vi "Tosca-Visual Display TCP Server.vi"(0 "Address":string, 7 "Port":i32, 11 "Queue":refnum<queue>) -> (15 "No Error":errorcluster)   [LabVIEW 2020]
uses:
  Tosca-Visual Display Queue Data.ctl
  Tosca-Visual Display Action.ctl
  Tosca-Grating.ctl
  Tosca-Grating Type.ctl
panel:
  out "date/time string":string
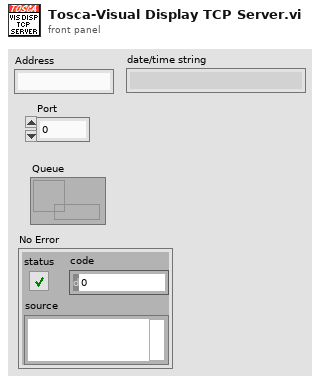
[diagram p1: front panel]
types:
  T1 = typedef "Tosca-Visual Display Queue Data.ctl" = cluster{"Action":T2, "Grating":T3}
  T2 = typedef "Tosca-Visual Display Action.ctl" = enum16{"NOOP", "Quit", "Buffer", "Draw", "Clear"}
  T3 = typedef "Tosca-Grating.ctl" = cluster{"Type":T4, "Orientation (deg)":dbl, "Spatial frequency (cpd)":dbl, "Velocity (Hz)":dbl, "Contrast":dbl, "Background intensity":dbl, "Duration (ms)":dbl, "Phase (cycles)":dbl}
  T4 = typedef "Tosca-Grating Type.ctl" = enum16{"OFF", "Square", "Sine"}
  T5 = cluster{"Grating type":T4, dbl, dbl, dbl, dbl, dbl, dbl, dbl}
  T6 = cluster{"Action":T2, cluster{"Grating type":T4, dbl, dbl, dbl, dbl, dbl, dbl, dbl}}
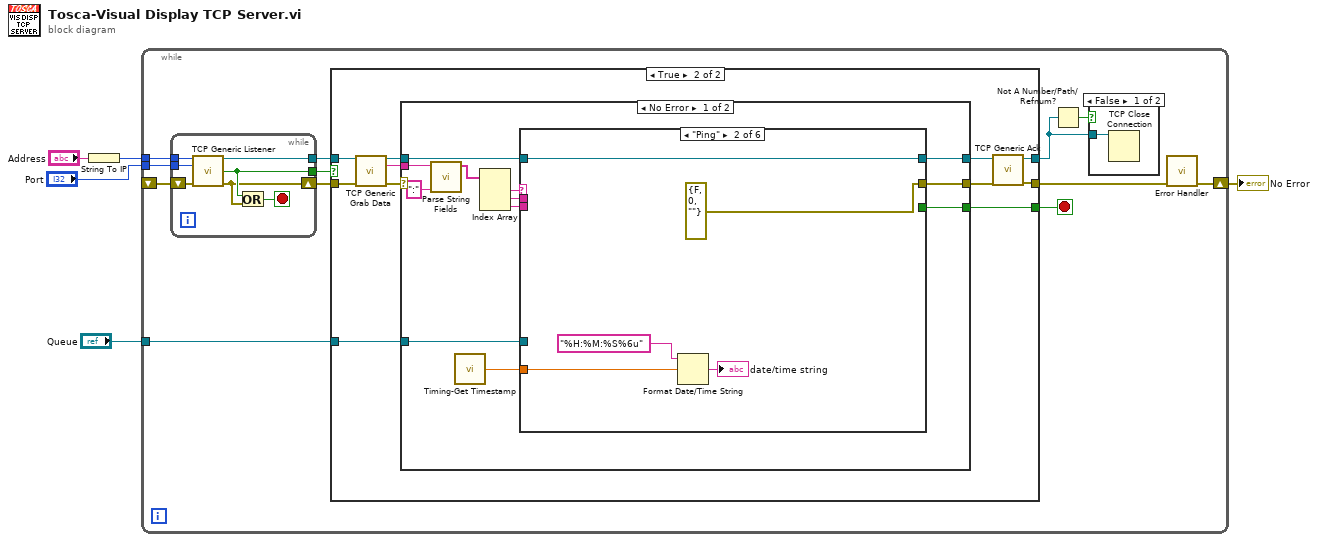
[diagram p0: block diagram]
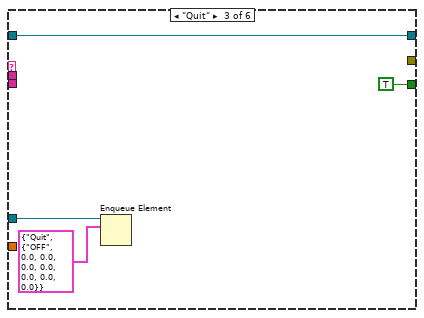
[diagram p5: hidden frame]
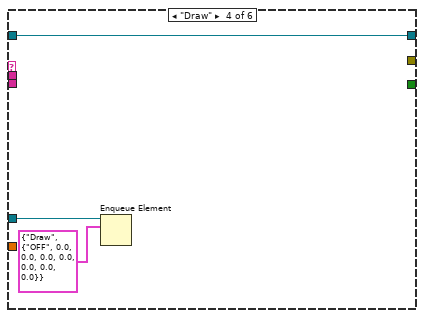
[diagram p6: hidden frame]
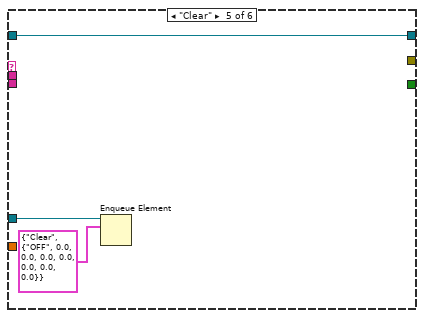
[diagram p7: hidden frame]
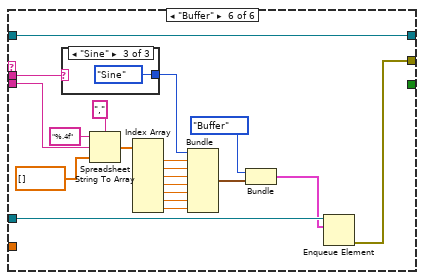
[diagram p8: hidden frame]
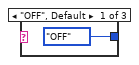
[diagram p9: hidden frame]
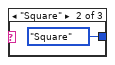
[diagram p10: hidden frame]
diagram:
  n1 = String To IP(1:"Address") -> (0:w4:u32)
  n2 = while {
    tunnel: w4 -> [w17]
    tunnel: "Port" -> [w16]
    shift-right: [w8] -> w2
    shift-left: _ -> [w15]
    tunnel: "Queue" -> [w6]
    stop <- w7 stop-if-true
    n3 = while {
      tunnel: w17 -> [w91]
      tunnel: w16 -> [w90]
      shift-right: [w86] -> w14
      shift-left: w15 -> [w89]
      tunnel: [w87] -> w13
      tunnel: [w88] -> w12
      stop <- w85 stop-if-true
      n4 = call "TCP Generic Listener.vi"("net address"=w91, "port"=w90, "error in (no error)"=w89) -> ("connection ID"=w88:refnum<k5>, "Connected?"=w87:bool, "error out"=w86:errorcluster)  [unwired: 10 in]
      n5 = Or(x=w87, y=w86) -> (x .or. y?=w85:bool)
    }
    n6 = case shown="True" w13 {
      tunnel: w14 -> [w19 w21]
      tunnel: w12 -> [w20 w31]
      tunnel: [w20 w25] -> w10
      tunnel: [w19 w24] -> w9
      tunnel: [_ w23] -> w7
      tunnel: w6 -> [_ w22]
      frame False {
      }
      frame True {
        n7 = call "TCP Generic Grab Data.vi"("connection ID"=w31, "error in (no error)"=w21) -> ("connection ID out"=w28:refnum<k5>, "data out"=w30:string, "error out"=w29:errorcluster)  [unwired: 11 in]
        n8 = case shown="No Error" w29 {
          selector: w29 -> [_ w83]
          tunnel: w30 -> [w43 _]
          tunnel: w28 -> [w42 w84]
          tunnel: [w39 w84] -> w27
          tunnel: [w38 w83] -> w26
          tunnel: [w37 _] -> w23
          tunnel: w22 -> [w33 _]
          frame No Error {
            n9 = call "Parse String Fields.vi"("Separator"=":", "String"=w43) -> ("Fields"=w41:string[])  [unwired: 8 in, 1 out]
            n10 = call "Timing-Get Timestamp.vi"() -> ("double precision float"=w32:dbl)  [unwired: 14 in, 1 out]
            n11 = Index Array(array=w41) -> (element #1=w40:string, element #2=w36:string, element #3=w35:string)  [unwired: 3 in]
            n12 = case shown="\"Ping\"" w40 {
              tunnel: w42 -> [w44 w49 w53 w56 w59 w79]
              tunnel: [w44 w49 w53 w56 w59 w79] -> w39
              tunnel: [_ errorcluster {"status"=FALSE, "code"=0, "source"=""} ("error constant") _ _ _ w77] -> w38
              tunnel: [_ _ TRUE _ _ _] -> w37
              tunnel: w36 -> [_ _ _ _ _ w73]
              tunnel: w35 -> [_ _ _ _ _ w76]
              tunnel: w33 -> [_ _ w51 w55 w58 w78]
              tunnel: w32 -> [_ w45 _ _ _ _]
              frame "", Default {
              }
              frame "Ping" {
                n13 = Format Date/Time String(time format string (%c)="%H:%M:%S%6u", seconds (now)=w45) -> (date/time string=→"date/time string":string)  [unwired: 1 in]
              }
              frame "Quit" {
                n14 = Enqueue Element(queue=w51, element=T1 {"Action"=enum."Quit", "Grating"={"Type"=enum."OFF", "Orientation (deg)"=0.0, "Spatial frequency (cpd)"=0.0, "Velocity (Hz)"=0.0, "Contrast"=0.0, "Background intensity"=0.0, "Duration (ms)"=0.0, "Phase (cycles)"=0.0}} ("Queue Data")) -> ()  [unwired: 2 in, 3 out]
              }
              frame "Draw" {
                n15 = Enqueue Element(queue=w55, element=T1 {"Action"=enum."Draw", "Grating"={"Type"=enum."OFF", "Orientation (deg)"=0.0, "Spatial frequency (cpd)"=0.0, "Velocity (Hz)"=0.0, "Contrast"=0.0, "Background intensity"=0.0, "Duration (ms)"=0.0, "Phase (cycles)"=0.0}} ("Queue Data")) -> ()  [unwired: 2 in, 3 out]
              }
              frame "Clear" {
                n16 = Enqueue Element(queue=w58, element=T1 {"Action"=enum."Clear", "Grating"={"Type"=enum."OFF", "Orientation (deg)"=0.0, "Spatial frequency (cpd)"=0.0, "Velocity (Hz)"=0.0, "Contrast"=0.0, "Background intensity"=0.0, "Duration (ms)"=0.0, "Phase (cycles)"=0.0}} ("Queue Data")) -> ()  [unwired: 2 in, 3 out]
              }
              frame "Buffer" {
                n17 = case shown="\"Sine\"" w73 {
                  tunnel: [Tosca-Grating_Type."OFF" ("Grating type") Tosca-Grating_Type."Square" ("Grating type") Tosca-Grating_Type."Sine" ("Grating type")] -> w70
                  frame "OFF", Default {
                  }
                  frame "Square" {
                  }
                  frame "Sine" {
                  }
                }
                n18 = Spreadsheet String To Array(delimiter (Tab)=",", format string="%.4f", spreadsheet string=w76, array type (2D Dbl)=dbl[] []) -> (array=w72:dbl[])
                n19 = Index Array(array=w72) -> (element #1=w69:dbl, element #2=w68:dbl, element #3=w67:dbl, element #4=w66:dbl, element #5=w65:dbl, element #6=w64:dbl, element #7=w60:dbl)  [unwired: 7 in]
                n20 = Bundle("Grating type"=w70, w69, w68, w67, w66, w65, w64, w60) -> (w63:T5)  [unwired: 1 in]
                n21 = Bundle("Action"=Tosca-Visual_Display_Action."Buffer", w63) -> (w61:T6)  [unwired: 1 in]
                n22 = Enqueue Element(queue=w78, element=w61) -> (error out=w77:errorcluster)  [unwired: 2 in, 2 out]
              }
            }
          }
          frame Error {
          }
        }
        n23 = call "TCP Generic Ack.vi"("error in (no error)"=w26, "connection ID"=w27) -> ("error out"=w24:errorcluster, "connection ID out"=w25:refnum<k5>)  [unwired: 8 in]
      }
    }
    n24 = Not A Number/Path/Refnum?(number/path/refnum=w10) -> (NaN/Path/Refnum?=w11:bool)
    n25 = case shown="False" w11 {
      tunnel: w10 -> [w18 _]
      frame False {
        n26 = TCP Close Connection(connection ID=w18) -> ()  [unwired: 2 in, 2 out]
      }
      frame True {
      }
    }
    n27 = call "Error Handler.vi"("error in (no error)"=w9) -> ("No Error"=w8:errorcluster)  [unwired: 12 in, 2 out]
  }
  "No Error" <- w2
